vi "History Add.vi"(8 "error in (no error)":errorcluster, 10 "History Record":T1, 11 "Connection Refnum":T2) -> (0 "error out":errorcluster, 3 "Connection Refnum":T2)   [LabVIEW 2011]
uses:
  SI.LIB/ODBC/SQL Controls/Connection Refnum.ctl
  History Record.ctl
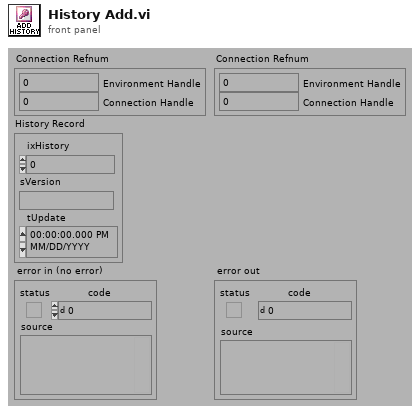
[diagram p1: front panel]
types:
  T1 = typedef "History Record.ctl" = cluster{"ixHistory":i32, "sVersion":string, "tUpdate":timestamp}
  T2 = typedef "Connection Refnum.ctl" = cluster{"Environment Handle":i32, "Connection Handle":i32}
  T3 = typedef "Statement Refnum.ctl" = cluster{"Statement Handle":i32, "Parameter Number":u16}
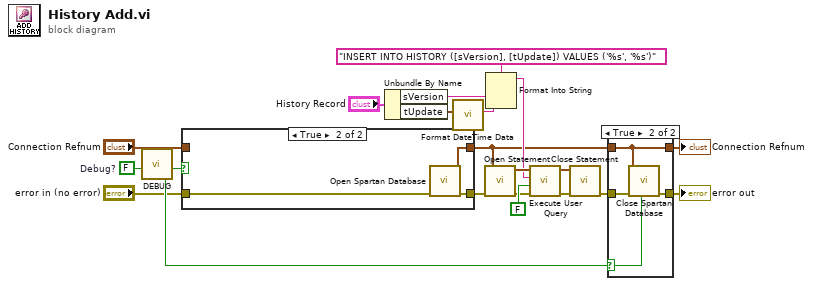
[diagram p0: block diagram]
diagram:
  w9 = FALSE  # Debug?
  n1 = call "DEBUG.vi"("Dev DEBUG? (f)"=w9) -> ("DEBUG?"=w8:bool)  [unwired: 1 in, 5 out]
  n2 = case shown="True" w8 {
    tunnel: "Connection Refnum" -> [w22 _]
    tunnel: "error in (no error)" -> [w21 w25]
    tunnel: [w21 w24] -> w4
    tunnel: [w22 w23] -> w1
    frame False {
    }
    frame True {
      n3 = call "Open Spartan Database.vi"("error in (no error)"=w25) -> ("error out"=w24:errorcluster, "Connection Refnum"=w23:T2)  [unwired: 2 in, 7 out]
    }
  }
  n4 = Unbundle By Name("History Record") -> ("sVersion"=w12:string, "tUpdate"=w11:timestamp)
  n5 = call "Format DateTime Data.vi"("Timestamp in"=w11) -> ("UTC DB String out"=w10:string)  [unwired: 10 out]
  n6 = call "Open Statement.vi"("error in (no error)"=w4, "Connection Refnum"=w1) -> ("error out"=w17:errorcluster, "Statement Refnum"=w16:T3)  [unwired: 4 out]
  n7 = Format Into String(format string="INSERT INTO HISTORY ([sVersion], [tUpdate]) VALUES ('%s', '%s')", w12, w10) -> (resulting string=w14:string)  [unwired: 2 in, 1 out]
  n8 = call "Execute User Query.vi"("error in (no error)"=w17, "Return Data? (f)"=FALSE, "User Query"=w14, "Statement Refnum"=w16) -> ("error out"=w18:errorcluster, "Statement Refnum"=w19:T3)  [unwired: 2 out]
  n9 = call "Close Statement.vi"("error in (no error)"=w18, "Statement Refnum"=w19) -> ("error out"=w2:errorcluster)  [unwired: 5 out]
  n10 = case shown="True" w8 {
    selector: w8 -> [_ w29]
    tunnel: w2 -> [w27 w31]
    tunnel: w1 -> [w26 w28]
    tunnel: [w26 w28] -> w3
    tunnel: [w27 w30] -> w7
    frame False {
    }
    frame True {
      n11 = call "Close Spartan Database.vi"("Force Close? (f)"=w29, "error in (no error)"=w31, "Connection Refnum"=w28) -> ("error out"=w30:errorcluster)  [unwired: 2 in, 6 out]
    }
  }
  "error out" <- w7
  "Connection Refnum" <- w3
